vi "Get Fault Statuses.vi"(4 "Fault String":string) -> (1 "Fault Descriptions":string)   [LabVIEW 2025, in "Interface Functions.lvlib"]
uses:
  Interface Functions.lvlib
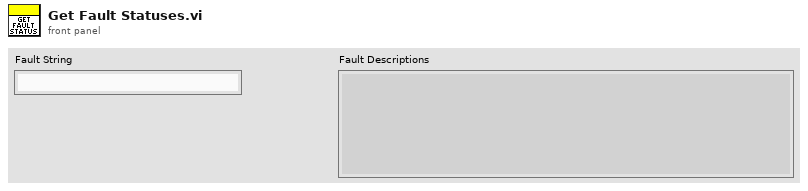
[diagram p1: front panel]
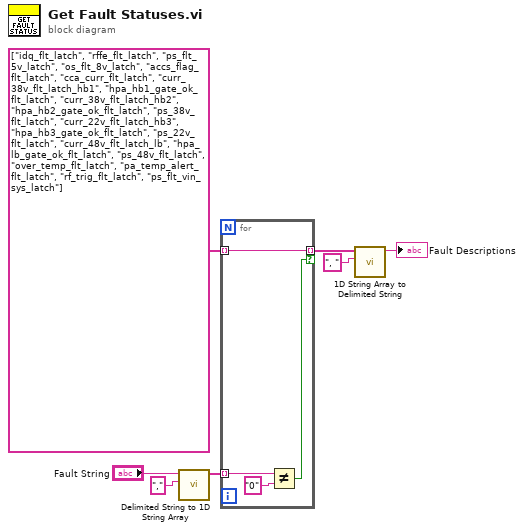
[diagram p0: block diagram]
diagram:
  n1 = call <vilib>:"Delimited String to 1D String Array.vi"("delimiter"=",", "delimited string"="Fault String") -> ("string array"=w5:string[])  [unwired: 9 in]
  n2 = for {
    tunnel: w5 -> [w11] mode=indexing
    tunnel: string[] ["idq_flt_latch", "rffe_flt_latch", "ps_flt_5v_latch", "os_flt_8v_latch", "accs_flag_flt_latch", "cca_curr_flt_latch", "curr_38v_flt_latch_hb1", "hpa_hb1_gate_ok_flt_latch", "curr_38v_flt_latch_hb2", "hpa_hb2_gate_ok_flt_latch", "ps_38v_flt_latch", "curr_22v_flt_latch_hb3", "hpa_hb3_gate_ok_flt_latch", "ps_22v_flt_latch", "curr_48v_flt_latch_lb", "hpa_lb_gate_ok_flt_latch", "ps_48v_flt_latch", "over_temp_flt_latch", "pa_temp_alert_flt_latch", "rf_trig_flt_latch", "ps_flt_vin_sys_latch"] -> [w9] mode=indexing
    tunnel: [w9] -> w3 mode=indexing if=w8
    n3 = Not Equal?(x=w11, y="0") -> (x != y?=w8:bool)
  }
  n4 = call <vilib>:"1D String Array to Delimited String.vi"("delimiter"=", ", "string array"=w3) -> ("delimited string"=→"Fault Descriptions":string)  [unwired: 9 in]
